vi "CS SQL Server.Listener.vi"() -> ()   [LabVIEW 2014, in "CS SQL Server.lvlib"]
doc: "This VI listens for connecting SQL clients and dispatches a SQL server for each.\nIt also monitors the the execution of SQL statements."
uses:
  CS SQL Server.lvlib
  CSlibraries/UtilityLib/UtilityLib.lvlib
panel:
  out "version":string
  out "Data Cluster":T1 {"SQL Input Cluster"."Version" format="%.2f"}
  out "#of open connections":i32
  out "SQL Server Port":u16=4711
  in  "stop":bool
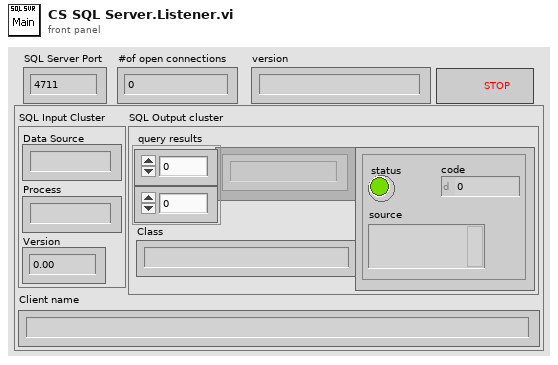
[diagram p1: front panel]
types:
  T1 = cluster{"SQL Input Cluster":cluster{"Data Source":string, "Process":string, "Version":dbl}, "SQL Output cluster":cluster{"query results":string[][], "Class":string, "error out":errorcluster}, "Client name":string}
  T2 = enum32{"invalid app kind", "Development System", "Run Time System", "Student Edition", "Embedded LabVIEW", "Evaluation", "Custom"}
  T3 = enum16{"add connection", "remove connection", "kill all connections", "default"}
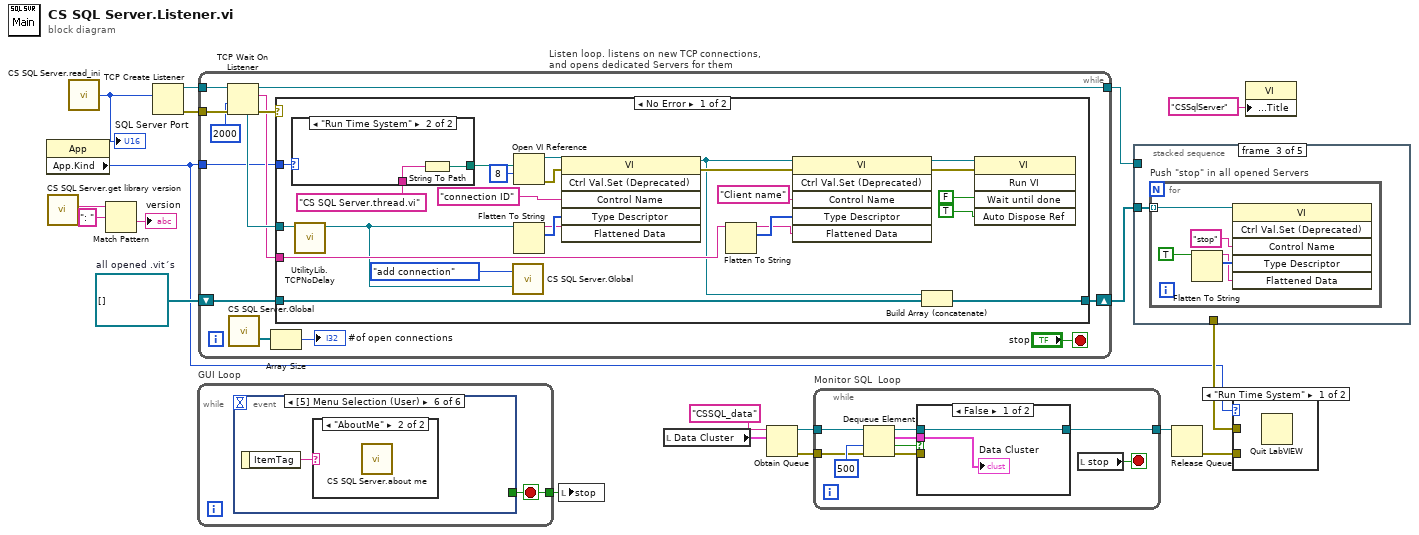
[diagram p0: block diagram]
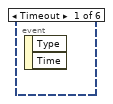
[diagram p2: hidden frame]
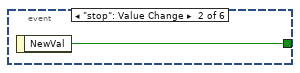
[diagram p3: hidden frame]
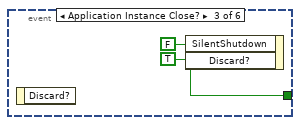
[diagram p4: hidden frame]
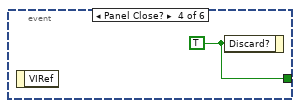
[diagram p5: hidden frame]
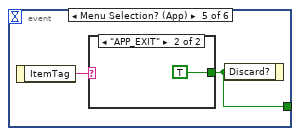
[diagram p6: hidden frame]
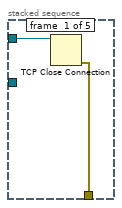
[diagram p10: hidden frame]
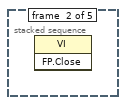
[diagram p11: hidden frame]
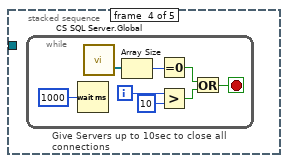
[diagram p12: hidden frame]
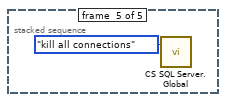
[diagram p13: hidden frame]
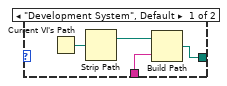
[diagram p15: hidden frame]
diagram:
  w11 = refnum<vi>[] []  # all opened .vit´s
  n1 = property class="App"() -> ("App.Kind"=w6:T2)  [unwired: 2 in, 2 out]
  n2 = call "CS SQL Server.get library version.vi"() -> ("nameAndVersion"=w4:string)  [unwired: 11 in]
  n3 = call "CS SQL Server.read_ini.vi"() -> ("Port"=w13:u32)
  "SQL Server Port" <- w13
  n4 = Match Pattern(string=w4, regular expression=": ") -> (after substring=→"version":string)  [unwired: 1 in, 3 out]
  n5 = TCP Create Listener(10:w13) -> (0:w19:errorcluster, 3:w18:refnum<k5>)  [unwired: 4 in, 1 out]
  n6 = while "GUI Loop" {
    tunnel: [w20] -> w1
    stop <- w20 stop-if-true
    n7 = event shown="[5] Menu Selection (User)" {
      selector: _ -> [_ _ _ _ _ _]
      dyn-events: _ -> [_ _ _ _ _ _]
      timeout: _ -> [_ _ _ _ _ _]
      tunnel: [_ w21 w22 w24 w25 _] -> w20
      event Timeout {
        n8 = event-data() -> ()  [unwired: 1 in, 2 out]
      }
      event "stop": Value Change {
        n9 = event-data() -> ("NewVal"=w21:bool)  [unwired: 1 in]
      }
      event Application Instance Close? {
        w22 = TRUE ("Discard?")
        n10 = event-data() -> ()  [unwired: 1 in, 1 out]
        n11 = event-data("SilentShutdown"=FALSE, "Discard?"=w22) -> ()  [unwired: 1 in, 1 out]
      }
      event Panel Close? {
        w24 = TRUE ("Discard?")
        n12 = event-data() -> ()  [unwired: 1 in, 1 out]
        n13 = event-data("Discard?"=w24) -> ()  [unwired: 1 in, 1 out]
      }
      event Menu Selection? (App) {
        n14 = event-data() -> ("ItemTag"=w26:string)  [unwired: 1 in]
        n15 = case shown="\"APP_EXIT\"" w26 {
          tunnel: [_ TRUE] -> w25
          frame "False", Default {
          }
          frame "APP_EXIT" {
          }
        }
        n16 = event-data("Discard?"=w25) -> ()  [unwired: 1 in, 1 out]
      }
      event Menu Selection (User) {
        n17 = event-data() -> ("ItemTag"=w28:string)  [unwired: 1 in]
        n18 = case shown="\"AboutMe\"" w28 {
          frame "False", Default {
          }
          frame "AboutMe" {
            n19 = call "CS SQL Server.about me.vi"() -> ()  [unwired: 1 in]
          }
        }
      }
    }
  }
  n20 = while "Listen loop. listens on new TCP connections, and opens dedicated Servers for them" {
    tunnel: w18 -> [w40]
    tunnel: w19 -> [w41]
    tunnel: [w38] -> w9
    shift-right: [w31] -> w10
    shift-left: w11 -> [w33]
    tunnel: w6 -> [w29]
    stop <- "stop" stop-if-true
    n21 = TCP Wait On Listener(8:w41, 9:2000, 11:w40) -> (0:w37:errorcluster, 2:w34:string, 3:w38:refnum<k5>, 4:w36:refnum<k5>)  [unwired: 1 in, 1 out]
    n22 = call "CS SQL Server.Global.vi"() -> ("Open Connections"=w30:refnum<k5>[])  [unwired: 19 in]
    n23 = Array Size(array=w30) -> (size(s)=→"#of open connections":i32)
    n24 = case shown="No Error" w37 {
      tunnel: w36 -> [w65 _]
      tunnel: w34 -> [w64 _]
      tunnel: w33 -> [w63 w72]
      tunnel: [w62 w72] -> w31
      tunnel: w29 -> [w44 _]
      frame No Error {
        n25 = case shown="\"Run Time System\"" w44 {
          tunnel: [w67 w70] -> w61
          tunnel: "CS SQL Server.thread.vi" ("Class") -> [w66 w71]
          frame "Development System", Default {
            n26 = Current VI's Path() -> (path=w69:path)
            n27 = Strip Path(path=w69) -> (stripped path=w68:path)  [unwired: 1 out]
            n28 = Build Path(base path=w68, name or relative path=w66) -> (appended path=w67:path)
          }
          frame "Run Time System" {
            n29 = String To Path(string=w71) -> (path=w70:path)
          }
        }
        n30 = call "UtilityLib.TCPNoDelay.vi"("connection in"=w65) -> ("connection out"=w45:refnum<k5>)  [unwired: 9 in, 1 out]
        n31 = call "CS SQL Server.Global.vi"("command"=T3."add connection", "connection"=w45) -> ()  [unwired: 17 in, 1 out]
        n32 = Open VI Reference(vi path=w61, options=8) -> (vi reference=w55:refnum<vi>, error out=w54:errorcluster)  [unwired: 4 in]
        n33 = Flatten To String(anything=w45) -> (data string=w58:string, type string=w59:i16[])  [unwired: 3 in, 1 out]
        n34 = invoke class="VI" method="Ctrl Val.Set (Deprecated)"(reference=w55, error in=w54, "Control Name"="connection ID", "Type Descriptor"=w59, "Flattened Data"=w58) -> (reference out=w47:refnum<vi>, error out=w53:errorcluster)  [unwired: 1 in, 4 out]
        n35 = Flatten To String(anything=w64) -> (data string=w48:string, type string=w49:i16[])  [unwired: 3 in, 1 out]
        n36 = invoke class="VI" method="Ctrl Val.Set (Deprecated)"(reference=w47, error in=w53, "Control Name"="Client name", "Type Descriptor"=w49, "Flattened Data"=w48) -> (reference out=w52:refnum<vi>, error out=w51:errorcluster)  [unwired: 1 in, 4 out]
        n37 = Build Array (concatenate)(w47, w63) -> (w62:refnum<vi>[])
        n38 = invoke class="VI" method="Run VI"(reference=w52, error in=w51, "Wait until done"=FALSE, "Auto Dispose Ref"=TRUE) -> ()  [unwired: 1 in, 5 out]
      }
      frame Error {
      }
    }
  }
  n39 = local write "stop"(w1) -> ()
  n40 = local read "Data Cluster"() -> (w12:T1)
  n41 = Obtain Queue(name (unnamed)="CSSQL_data", element data type=w12) -> (queue out=w15:refnum<queue>, error out=w14:errorcluster)  [unwired: 3 in, 1 out]
  n42 = while "Monitor SQL  Loop" {
    tunnel: w15 -> [w80]
    tunnel: w14 -> [w75]
    tunnel: [w76] -> w17
    stop <- w81 stop-if-true
    n43 = Dequeue Element(queue=w80, timeout in ms (-1)=500, error in (no error)=w75) -> (queue out=w77:refnum<queue>, element=w73:T1, timed out?=w79:bool, error out=w74:errorcluster)
    n44 = case shown="False" w79 {
      tunnel: w77 -> [w83 w84]
      tunnel: [w83 w84] -> w76
      tunnel: w74 -> [_ _]
      tunnel: w73 -> [w82 _]
      frame False {
        "Data Cluster" <- w82
      }
      frame True {
      }
    }
    n45 = local read "stop"() -> (w81:bool)
  }
  n46 = stacked-sequence {
    tunnel: w10 -> [_ _ w87 _ _]
    tunnel: w9 -> [w86 _ _ _ _]
    tunnel: [w85 _ _ _ _] -> w8
    frame #0 {
      n47 = TCP Close Connection(connection ID=w86) -> (error out=w85:errorcluster)  [unwired: 2 in, 1 out]
    }
    frame #1 {
      n48 = invoke class="VI" method="FP.Close"() -> ()  [unwired: 3 in, 3 out]
    }
    frame #2 {
      n49 = for "Push \"stop\" in all opened Servers" {
        tunnel: w87 -> [w88] mode=indexing
        n50 = Flatten To String(anything=TRUE) -> (data string=w89:string, type string=w90:i16[])  [unwired: 3 in, 1 out]
        n51 = invoke class="VI" method="Ctrl Val.Set (Deprecated)"(reference=w88, "Control Name"="stop", "Type Descriptor"=w90, "Flattened Data"=w89) -> ()  [unwired: 2 in, 6 out]
      }
    }
    frame #3 {
      n52 = while "Give Servers up to 10sec to close all connections" {
        i -> [w98]
        stop <- w94 stop-if-true
        n53 = Wait (ms)(milliseconds to wait=u32 1000) -> ()  [unwired: 1 out]
        n54 = call "CS SQL Server.Global.vi"() -> ("Open Connections"=w100:refnum<k5>[])  [unwired: 19 in]
        n55 = Array Size(array=w100) -> (size(s)=w99:i32)
        n56 = Equal To 0?(x=w99) -> (x = 0?=w97:bool)
        n57 = Greater?(x=w98, y=10) -> (0:w96:bool)
        n58 = Or(x=w97, y=w96) -> (x .or. y?=w94:bool)
      }
    }
    frame #4 {
      n59 = call "CS SQL Server.Global.vi"("command"=T3."kill all connections") -> ()  [unwired: 18 in, 1 out]
    }
  }
  n60 = Release Queue(queue=w17) -> (error out=w7:errorcluster)  [unwired: 2 in, 2 out]
  n61 = case shown="\"Run Time System\"" w6 {
    tunnel: w8 -> [_ _]
    tunnel: w7 -> [_ _]
    frame "Run Time System" {
      n62 = Quit LabVIEW() -> ()  [unwired: 1 in]
    }
    frame Default {
    }
  }
  n63 = property class="VI"("Front Panel.Title"="CSSqlServer" ("Front Panel Window:Title")) -> ()  [unwired: 2 in, 2 out]
